vi "Close MeasurementLink Session.vi"(8 "error in":errorcluster, 9 "initialize and close session behavior":T1, 10 "session in":variant, 11 "KeysightDmm in":refnum<class "KeysightDmm.lvclass">) -> (0 "error out":errorcluster)   [LabVIEW 2021, in "KeysightDmm.lvclass"]
doc: "Closes the local session. If the session represents a remote session, <b>initialize and close session behavior</b> determines whether closing the local session closes the server session or detaches from the server session."
uses:
  KeysightDmm.lvclass
  <vilib>/Plug-In SDKs/Sessions/Instrument/ISession Factory/Initialize and Close Session Behavior.ctl
  KeysightDmm.lvclass/KeysightDmm.ctl
  <instrlib>/Agilent 34401/Public/Close.vi
  <instrlib>/Agilent 34401/Agilent 34401.lvlib
  <vilib>/Plug-In SDKs/Sessions/Instrument/ISession Factory/ISession Factory.lvclass
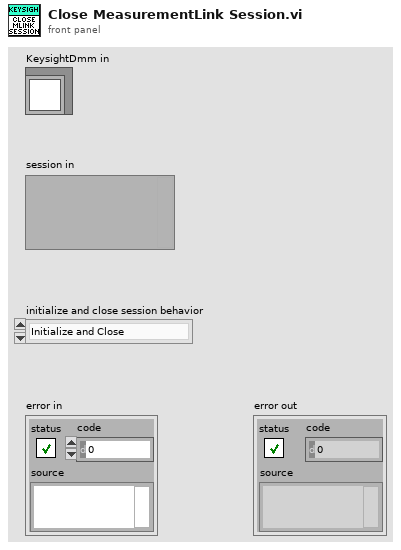
[diagram p1: front panel]
types:
  T1 = typedef "NI Session Management Instrument.lvlib/ISession Factory.lvclass/Initialize and Close Session Behavior.ctl" = enum16{"Initialize and Close", "Attach and Detach", "Initialize and Detach", "Attach and Close"}
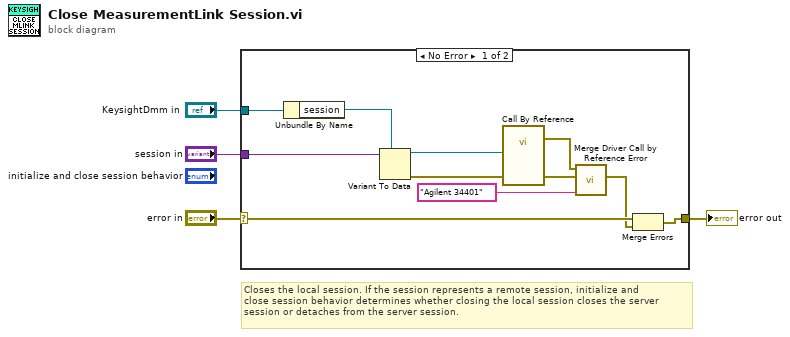
[diagram p0: block diagram]
diagram:
  # "Closes the local session. If the session represents a remote session, initialize and \nclose session behavior determines whether closing the local session closes the server \nsession or detaches from the server session."
  n1 = case shown="No Error" "error in" {
    selector: "error in" -> [w15 w16]
    tunnel: [w9 w16] -> w3
    tunnel: "session in" -> [w7 _]
    tunnel: "KeysightDmm in" -> [w6 _]
    frame No Error {
      n2 = Unbundle By Name(w6) -> ("session"=w5:refnum<visa-resource-name>)
      n3 = Variant To Data(type=w5, Variant=w7) -> (data=w10:refnum<visa-resource-name>, error out=w11:errorcluster)  [unwired: 1 in]
      n4 = call-by-ref "?"("error in (no error)"=w11, "VISA resource name"=w10) -> (error out=w13:errorcluster, 0:"error out"=w12:errorcluster)  [unwired: 11 in, 1 out]
      n5 = call <vilib>:"Merge Driver Call by Reference Error.vi"("driver name"="Agilent 34401", "called vi error"=w12, "call by ref error"=w13) -> ("error out"=w8:errorcluster)  [unwired: 8 in]
      n6 = Merge Errors(w15, w8) -> (w9:errorcluster)
    }
    frame Error {
    }
  }
  "error out" <- w3
